vi "Main.vi"() -> ()   [LabVIEW 2014]
panel:
  in  "stop loop 2":bool
  in  "Variant Selector":enum16{"Boolean", "Numeric", "String"}(ring)
  out "StringOut":string
  out "NumericOut":dbl
  out "BooleanOut":bool
  in  "StringIn":string
  in  "NumericIn":dbl
  in  "BooleanIn":bool
  in  "stop loop 1":bool
  # "In"
  # "Out"
  # "Boolean\nVariant"
  # "Numeric\nVariant"
  # "String\nVariant"
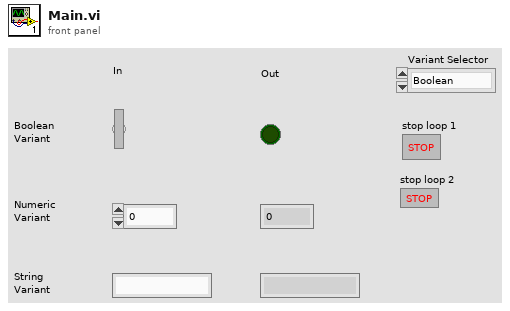
[diagram p1: front panel]
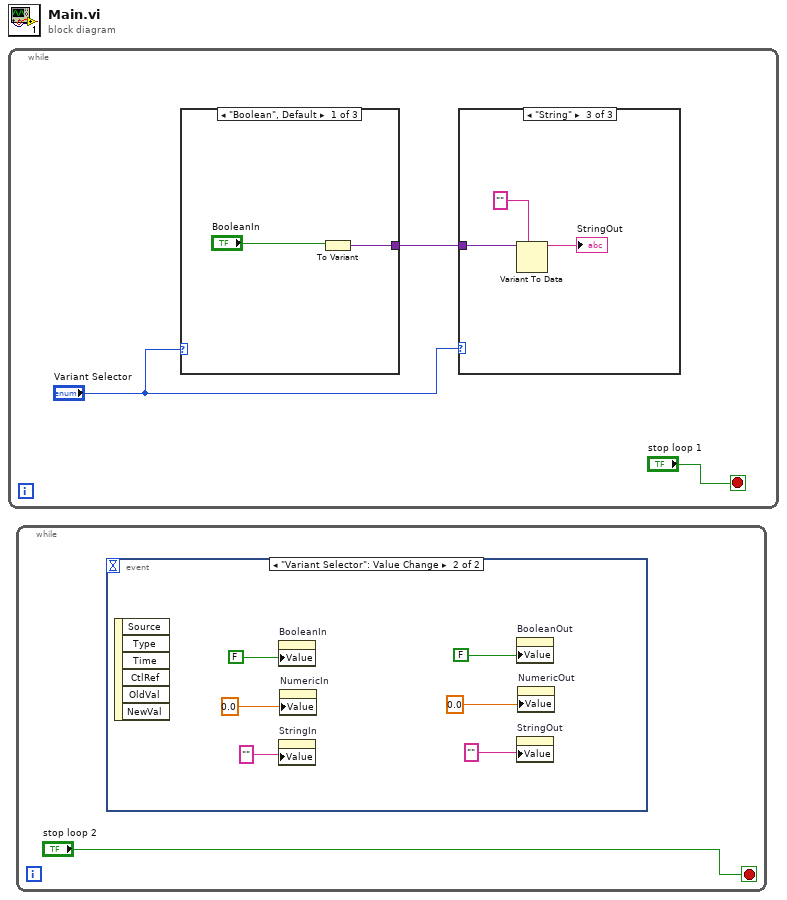
[diagram p0: block diagram]
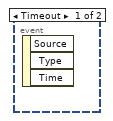
[diagram p2: hidden frame]
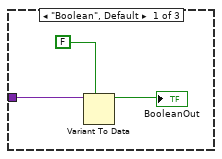
[diagram p3: hidden frame]
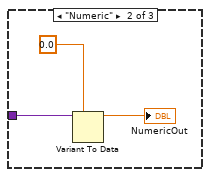
[diagram p4: hidden frame]
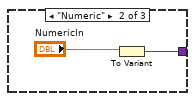
[diagram p5: hidden frame]
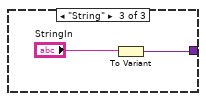
[diagram p6: hidden frame]
diagram:
  n1 = while {
    stop <- "stop loop 1" stop-if-true
    n2 = case shown="\"Boolean\", Default" "Variant Selector" {
      tunnel: [w14 w16 w17] -> w3
      frame "Boolean", Default {
        n3 = To Variant(anything="BooleanIn") -> (Variant=w14:variant)
      }
      frame "Numeric" {
        n4 = To Variant(anything="NumericIn") -> (Variant=w16:variant)
      }
      frame "String" {
        n5 = To Variant(anything="StringIn") -> (Variant=w17:variant)
      }
    }
    n6 = case shown="\"String\"" "Variant Selector" {
      tunnel: w3 -> [w6 w9 w12]
      frame "Boolean", Default {
        n7 = Variant To Data(type=FALSE, Variant=w6) -> (data=→"BooleanOut":bool)  [unwired: 1 in, 1 out]
      }
      frame "Numeric" {
        n8 = Variant To Data(type=0.0, Variant=w9) -> (data=→"NumericOut":dbl)  [unwired: 1 in, 1 out]
      }
      frame "String" {
        n9 = Variant To Data(type="", Variant=w12) -> (data=→"StringOut":string)  [unwired: 1 in, 1 out]
      }
    }
  }
  n10 = while {
    stop <- "stop loop 2" stop-if-true
    n11 = event shown="[1] \"Variant Selector\": Value Change" {
      selector: _ -> [_ _]
      dyn-events: _ -> [_ _]
      timeout: _ -> [_ _]
      event Timeout {
        n12 = event-data() -> ()  [unwired: 1 in, 3 out]
      }
      event "Variant Selector": Value Change {
        n13 = event-data() -> ()  [unwired: 1 in, 6 out]
        n14 = property on="BooleanIn" class="Bool (strict)"("Value"=FALSE) -> ()  [unwired: 2 in, 2 out]
        n15 = property on="StringIn" class="Str"("Value"="" ("StringIn")) -> ()  [unwired: 2 in, 2 out]
        n16 = property on="NumericIn" class="DigNum (strict)"("Value"=0.0 ("NumericIn")) -> ()  [unwired: 2 in, 2 out]
        n17 = property on="BooleanOut" class="Bool (strict)"("Value"=FALSE) -> ()  [unwired: 2 in, 2 out]
        n18 = property on="StringOut" class="Str"("Value"="" ("StringIn")) -> ()  [unwired: 2 in, 2 out]
        n19 = property on="NumericOut" class="DigNum (strict)"("Value"=0.0 ("NumericIn")) -> ()  [unwired: 2 in, 2 out]
      }
    }
  }
